vi "Write sampling info.vi"(8 "error in (no error)":errorcluster, 10 "sampling info":cluster{"Fs":dbl, "#s":u32}={"Fs"=1000.0, "#s"=1000} {"Fs" format="%.2p"}, 11 "LockinDAQ in":refnum<class "LockinDAQ.lvclass">) -> (0 "error out":errorcluster, 3 "LockinDAQ out":refnum<class "LockinDAQ.lvclass">)   [LabVIEW 2016, in "LockinDAQ.lvclass"]
uses:
  LockinDAQ.lvclass
  LockinDAQ.lvclass/LockinDAQ.ctl
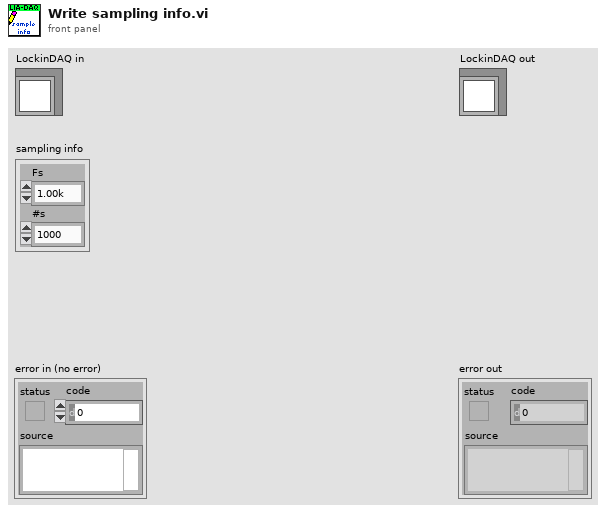
[diagram p1: front panel]
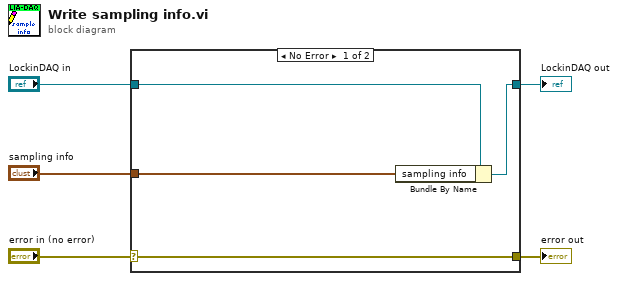
[diagram p0: block diagram]
diagram:
  n1 = case shown="No Error" "error in (no error)" {
    selector: "error in (no error)" -> [w9 w10]
    tunnel: [w9 w10] -> w4
    tunnel: [w7 w11] -> w2
    tunnel: "LockinDAQ in" -> [w8 w11]
    tunnel: "sampling info" -> [w6 _]
    frame No Error {
      n2 = Bundle By Name(cluster=w8, "sampling info"=w6) -> (w7:refnum<class "LockinDAQ.lvclass">)
    }
    frame Error {
    }
  }
  "error out" <- w4
  "LockinDAQ out" <- w2
